vi "Bundler Test.vi"() -> ()   [LabVIEW 2020]
panel:
  out "output cluster":cluster{"Bool":bool, "String":string}
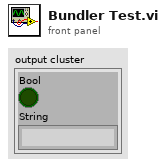
[diagram p1: front panel]
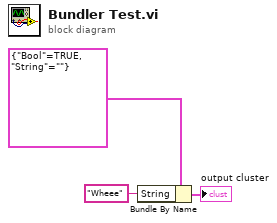
[diagram p0: block diagram]
diagram:
  n1 = Bundle By Name(cluster=cluster{"Bool":bool, "String":string} {"Bool"=TRUE, "String"=""}, "String"="Wheee") -> (→"output cluster":cluster{"Bool":bool, "String":string})
